vi "niScope Configure Trigger Digital.vi"(0 "instrument handle":refnum<k15>, 1 "trigger slope":T2, 5 "trigger source":T1="VAL_RTSI_0", 11 "error in":errorcluster, 12 "trigger holdoff":dbl format="%.4f", 13 "trigger delay":dbl format="%.4f") -> (4 "instrument handle out":refnum<k15>, 15 "error out":errorcluster)   [LabVIEW 2011]
doc: "Configures the common properties of a digital trigger."
uses:
  <instrlib>/niScope/Controls/niScope trigger slope.ctl
  <instrlib>/niScope/Controls/niScope trigger source digital.ctl
  niScope_32.dll
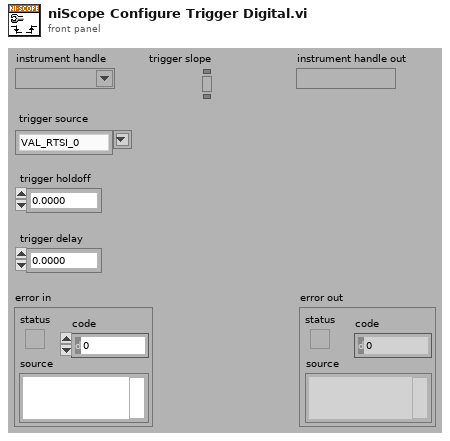
[diagram p1: front panel]
types:
  T1 = typedef "niScope trigger source digital.ctl" = string
  T2 = typedef "niScope trigger slope.ctl" = i32
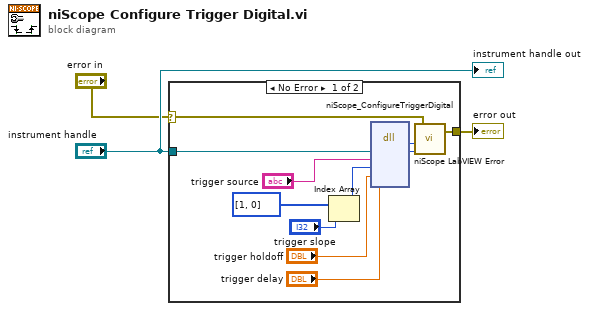
[diagram p0: block diagram]
diagram:
  n1 = case shown="No Error" "error in" {
    selector: "error in" -> [w5 w15]
    tunnel: [w11 w15] -> w3
    tunnel: "instrument handle" -> [w14 _]
    frame No Error {
      n2 = Index Array(array=i32[] [1, 0] ("trigger slope arr"), index="trigger slope") -> (element=w8:i32)
      n3 = dll-call lib="niScope_*.*" fn="niScope_ConfigureTriggerDigital"("instrument handle"=w14, "triggerSource"="trigger source", "slope"=w8, "holdoff"="trigger holdoff", "delay"="trigger delay") -> ("status"=w13:i32, "instrument handle"=w12:u32)  [unwired: 7 in, 2 out]
      n4 = call <instrlib>:"niScope LabVIEW Error.vi"("instrument handle"=w12, "niScope error code (0)"=w13, "error in (no error)"=w5) -> ("error out"=w11:errorcluster)  [unwired: 2 in]
    }
    frame Error {
    }
  }
  "error out" <- w3
  "instrument handle out" <- "instrument handle"
